vi "ROI entry screen-LBox create text.vi"(8 "error in (no error)":errorcluster) -> (0 "error out":errorcluster, 3 "Array":string[][](array[string]))   [LabVIEW 2020]
uses:
  Typedefs/ROI management FG states.ctl
  Globals/gl_ROI Entry UI globals.vi
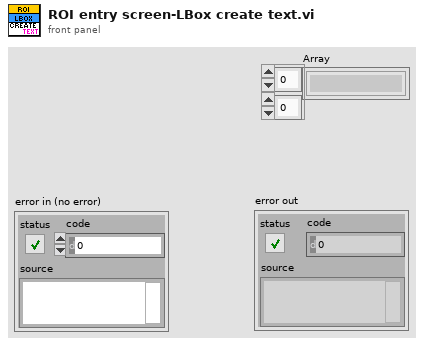
[diagram p1: front panel]
types:
  T1 = typedef "ROI management FG states.ctl" = enum16{"Read", "Write", "Write-from dataset", "Clear Last", "Clear All", "Delete ROI", "Update ROIs time", "Reload last ROI set", "Modify ROI Parameters", "Offset all ROI", "Offset visible ROI", "Modify Dwell Time", "Modify Laser Power"}
  T2 = typedef "ROI entry screen ctrl refs cluster.ctl" = cluster{"Done button":refnum<vi>, "Imaging button":refnum<vi>, "Acquisition button":refnum<vi>, "Scan dwell time per pixel (us)":refnum<vi>, "# of planes":refnum<vi>, "Zoom Ctrl":refnum<vi>, "Equal size":refnum<vi>, "Channel":refnum<vi>, "Image Display":refnum<vi>, "Z-Plane Selector":refnum<vi>, "Number of lines left":refnum<vi>, "Z-stack folder path":refnum<vi>, "POI Density":refnum<vi>, "Arb Plane Entry":refnum<vi>, "Whole Plane":refnum<vi>, "Line Mode":refnum<vi>, "Clear Last":refnum<vi>, "Clear All":refnum<vi>, "Delete Lines":refnum<vi>, "Trial Length (sec)":refnum<vi>, "Palette Type":refnum<vi>, "Intensity slider":refnum<vi>, "# POI":refnum<vi>, "Max Z Proj":refnum<vi>, "Zplane ind":refnum<vi>, "Wavelength (nm)":refnum<vi>, "Number of Trials":refnum<vi>, "Funct stim.trig.enable":refnum<vi>, "Funct stim.trig.delay (s)":refnum<vi>, "Line Mode":refnum<vi>, "Step size (µm)":refnum<vi>, "ROI move mode":refnum<vi>, "Cool-down time (s)":refnum<vi>, "Enable cool-down time":refnum<vi>, "Motor Z ind. (um)":refnum<vi>, "AOL Z ind. (um)":refnum<vi>, "Load Reference Image":refnum<vi>, "Rel.  Res.":refnum<vi>, "ROI LIST":refnum<vi>, "Show All":refnum<vi>, "ROI Type":refnum<vi>, "Start Plane":refnum<vi>, "Stop Plane":refnum<vi>, "Offset ROI":refnum<vi>, "Tab Control":refnum<vi>, "Laser Power(%)":refnum<vi>, "Cycle rate":refnum<vi>, "FOV (Ind.)":refnum<vi>, "Frame Size (Ind.)":refnum<vi>, "Resolution (Ind.)":refnum<vi>, "Pixel Density (Ind)":refnum<vi>, "Laser Power (Ind.)":refnum<vi>, "Dwell Time (Ind.)":refnum<vi>, "Adj MC":refnum<vi>}
  T3 = typedef "ROI parameters data type.ctl" = cluster{"ROI index":dbl, "ROI ID":dbl, "ROI Time (ns)":dbl, "Pixels in ROI":dbl, "X start":dbl, "Y start":dbl, "Z start":dbl, "X stop":dbl, "Y stop":dbl, "Z stop":dbl, "Angle (deg)":dbl, "Composite ID":dbl, "Number of lines":dbl, "Frame Size":dbl, "Zoom":dbl, "Laser Power (%)":dbl, "ROI group ID":dbl, "Resolution":dbl, "Dwell Time per pixel":dbl, "Pixels per miniscan":dbl, "Original FOV (um)":dbl, "Apparent Frame Size":dbl, "Z Plane Idx":i32[], "Z Plane codes":i32[]}
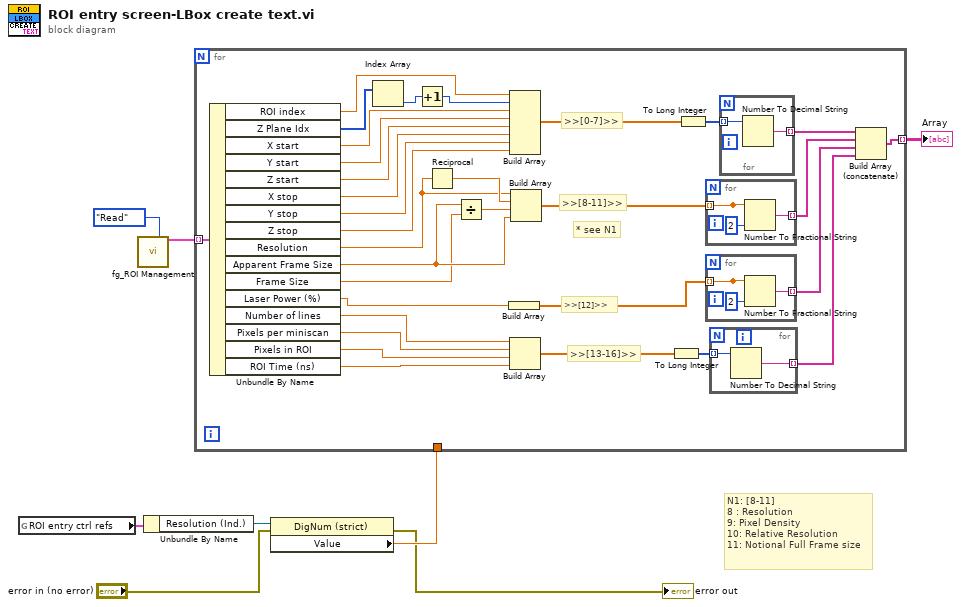
[diagram p0: block diagram]
diagram:
  # "N1: [8-11]\n8 : Resolution\n9: Pixel Density\n10: Relative Resolution\n11: Notional Full Frame size"
  n1 = global read "gl_ROI Entry UI globals.vi" "ROI entry ctrl refs"() -> (w5:T2)
  n2 = call "fg_ROI Management.vi"("Function"=ROI_management_FG_states."Read") -> ("ROI Setup"=w8:T3[])  [unwired: 8 in, 6 out]
  n3 = Unbundle By Name(w5) -> ("Resolution (Ind.)"=w4:refnum<vi>)
  n4 = property class="DigNum (strict)"(reference=w4, error in="error in (no error)") -> (error out=→"error out":errorcluster, "Value"=w3:dbl)  [unwired: 1 out]
  n5 = for {
    tunnel: w8 -> [w40] mode=indexing
    tunnel: [w23] -> w6 mode=indexing
    tunnel: w3 -> [_]
    # "* see N1"
    # ">>[13-16]>>"
    # ">>[12]>>"
    # ">>[8-11]>>"
    # ">>[0-7]>>"
    n6 = Unbundle By Name(w40) -> ("ROI index"=w31:dbl, "Z Plane Idx"=w32:i32[], "X start"=w39:dbl, "Y start"=w38:dbl, "Z start"=w37:dbl, "X stop"=w36:dbl, "Y stop"=w35:dbl, "Z stop"=w34:dbl, "Resolution"=w12:dbl, "Apparent Frame Size"=w11:dbl, "Frame Size"=w10:dbl, "Laser Power (%)"=w16:dbl, "Number of lines"=w27:dbl, "Pixels per miniscan"=w18:dbl, "Pixels in ROI"=w26:dbl, "ROI Time (ns)"=w25:dbl)
    n7 = Index Array(array=w32) -> (element=w20:i32)  [unwired: 1 in]
    n8 = Increment(x=w20) -> (x+1=w19:i32)
    n9 = Reciprocal(x=w12) -> (1/x=w17:dbl)
    n10 = Divide(x=w11, y=w10) -> (x/y=w9:dbl)
    n11 = Build Array(w16) -> (w15:dbl[])
    n12 = Build Array(w31, w19, w39, w38, w37, w36, w35, w34) -> (w33:dbl[])
    n13 = Build Array(w27, w18, w26, w25) -> (w24:dbl[])
    n14 = Build Array(w12, w17, w9, w11) -> (w29:dbl[])
    n15 = To Long Integer(number=w24) -> (32bit integer=w28:i32[])
    n16 = To Long Integer(number=w33) -> (32bit integer=w30:i32[])
    n17 = for {
      tunnel: [w47] -> _ mode=indexing
      tunnel: [w48] -> w21 mode=indexing
      tunnel: w29 -> [w47] mode=indexing
      n18 = Number To Fractional String(number=w47, precision (6)=i16 2) -> (F-format string=w48:string)  [unwired: 2 in]
    }
    n19 = for {
      tunnel: w15 -> [w42] mode=indexing
      tunnel: [w43] -> w14 mode=indexing
      tunnel: [w42] -> _ mode=indexing
      n20 = Number To Fractional String(number=w42, precision (6)=i16 2) -> (F-format string=w43:string)  [unwired: 2 in]
    }
    n21 = for {
      tunnel: w28 -> [w45] mode=indexing
      tunnel: [w44] -> w13 mode=indexing
      n22 = Number To Decimal String(number=w45) -> (decimal integer string=w44:string)  [unwired: 1 in]
    }
    n23 = for {
      tunnel: w30 -> [w50] mode=indexing
      tunnel: [w49] -> w22 mode=indexing
      n24 = Number To Decimal String(number=w50) -> (decimal integer string=w49:string)  [unwired: 1 in]
    }
    n25 = Build Array (concatenate)(w22, w21, w14, w13) -> (w23:string[])
  }
  "Array" <- w6
